vi "Example_Simple Acquire.vi"() -> ()   [LabVIEW 2015, in "G 5.lvlib"]
uses:
  <instrlib>/G 5.lvlib
  <vilib>/Utility/file.llb/Write To Spreadsheet File (DBL).vi
panel:
  in  "Display Duration [sec]":dbl=10.0
  in  "Acquisition Rate [Hz]":i16(ring)=2000 items=["10"=10, "15"=15, "20"=20, "25"=25, "30"=30, "40"=40, "45"=45, "50"=50, "60"=60, "75"=75, "80"=80, "90"=90, "100"=100, "120"=120, "125"=125, "150"=150, "180"=180, "200"=200, "225"=225, "240"=240, "250"=250, "300"=300, "360"=360, "400"=400, "450"=450, "500"=500, "600"=600, "800"=800, "900"=900, "1000"=1000, "1200"=1200, "1500"=1500, "1800"=1800, "2000"=2000]
  in  "Save Data":bool
  in  "Start Acquisition":bool
  in  "stop":bool
  in  "ZERO":bool
  in  "Gen 5":i32=1 min=1 step=1
  in  "CAPTURE":bool
  out "STATUS":bool=TRUE
  in  "Channel":i32=3
  in  "Value":dbl=5.0
  in  "Time [sec]":dbl=0.5 step=0.1 format="%.2g"
  out "Output Graph 2":waveform(dbl)[](graph)
  in  "Gen 5 Displayed 2":i64=2
  out "Output Graph 1":waveform(dbl)[](graph)
  in  "Gen 5 Displayed 1":i64=1
  # "TRIGGER CONTROL"
  # "ACQUISITION SETUP"
  # "ACQUISITION CONTROL"
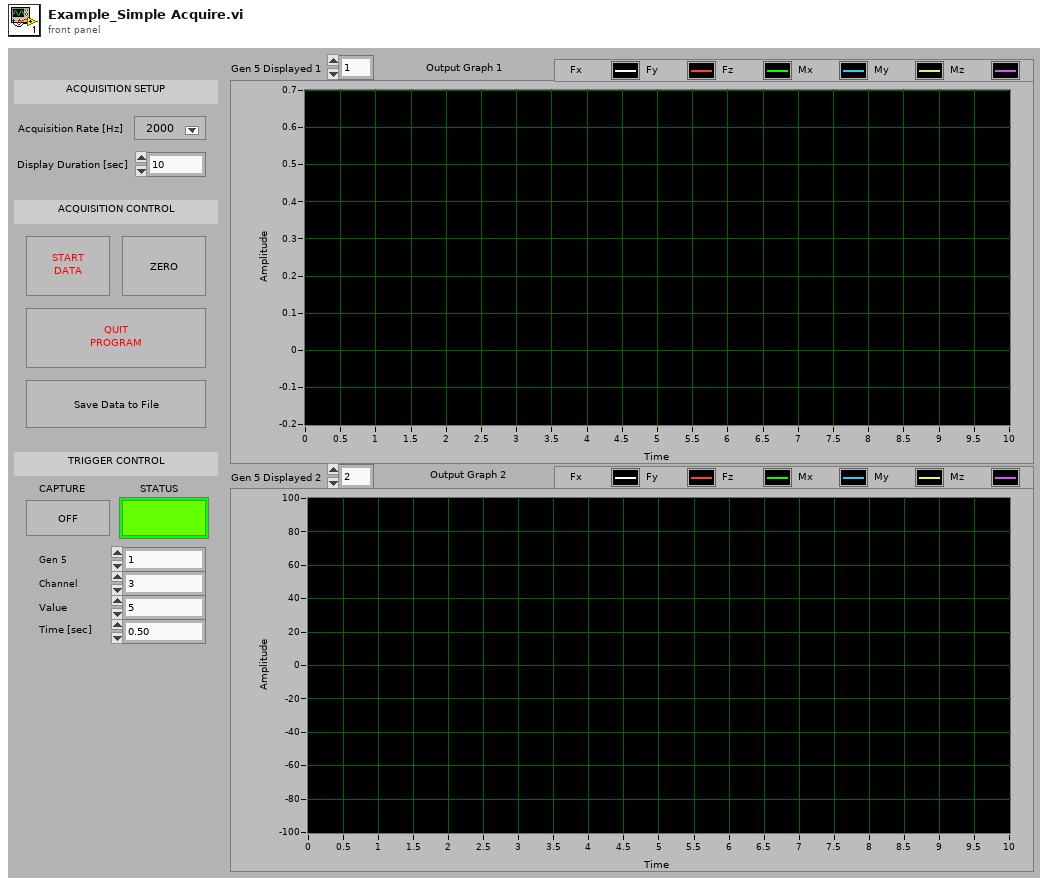
[diagram p1: front panel]
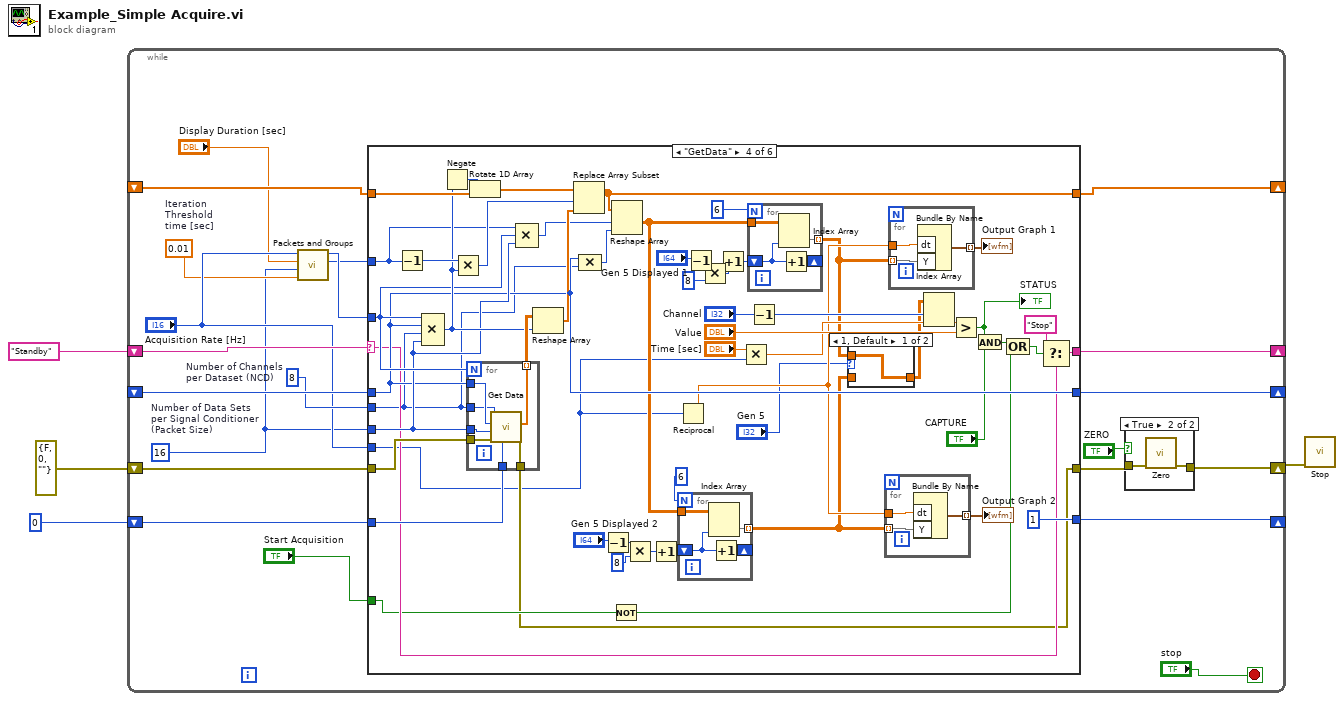
[diagram p0: block diagram]
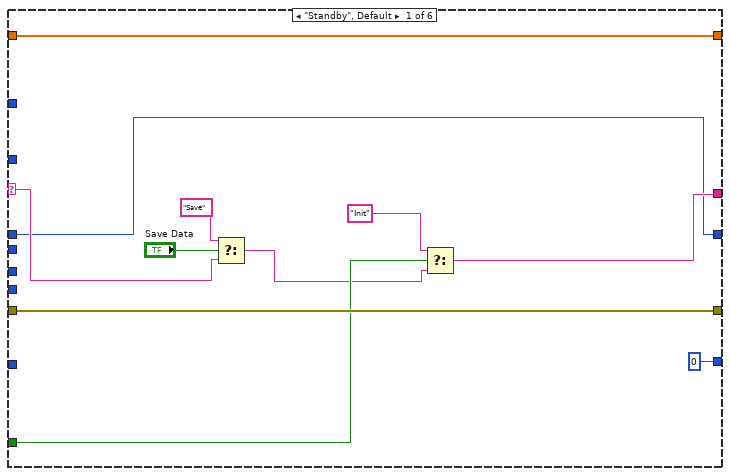
[diagram p3: hidden frame]
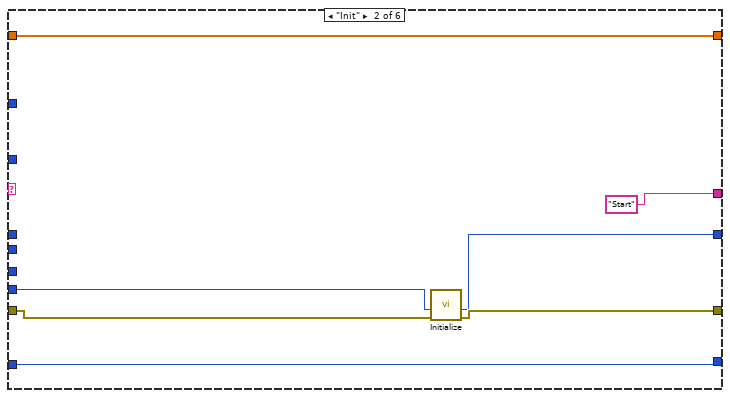
[diagram p4: hidden frame]
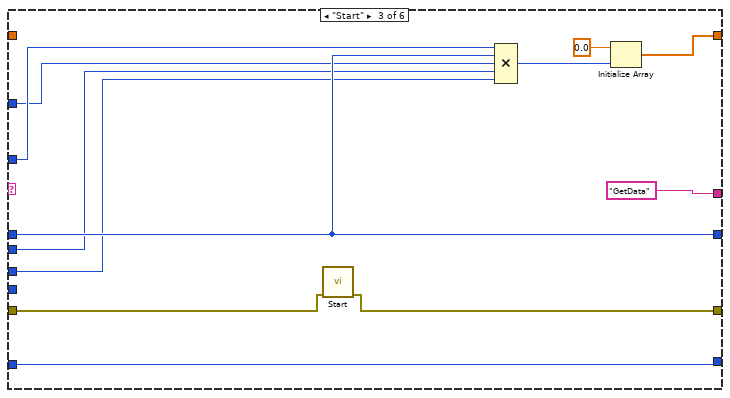
[diagram p5: hidden frame]
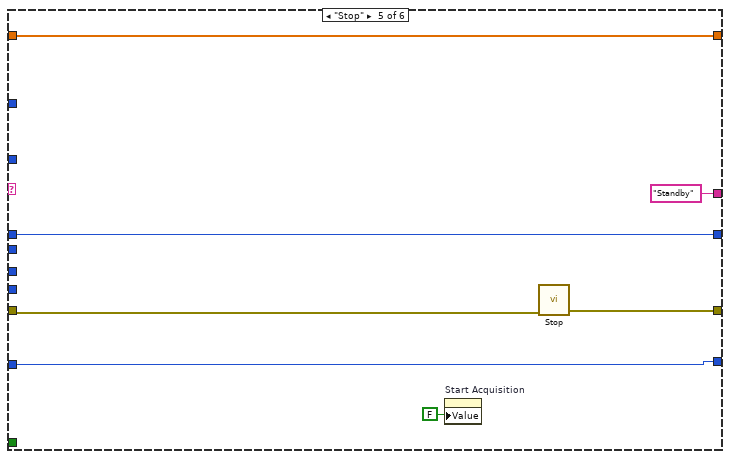
[diagram p7: hidden frame]
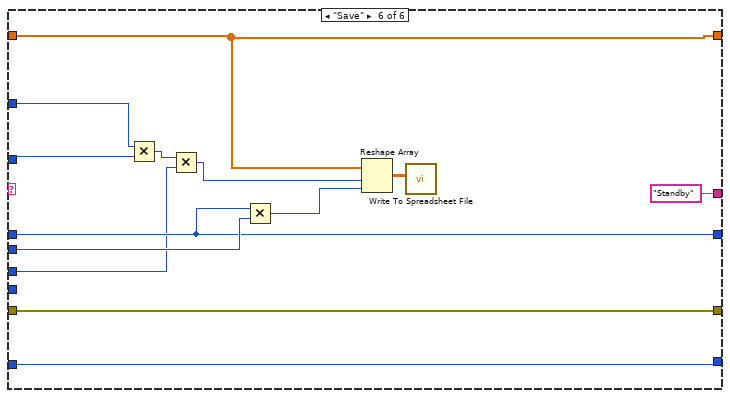
[diagram p8: hidden frame]
diagram:
  n1 = while {
    shift-right: [w20] -> _
    shift-left: "Standby" -> [w25]
    shift-right: [w23] -> w1
    shift-left: errorcluster {"status"=FALSE, "code"=0, "source"=""} ("error out") -> [w22]
    shift-right: [w19] -> _
    shift-left: _ -> [w18]
    shift-right: [w16] -> _
    shift-left: 0 -> [w17]
    shift-right: [w13] -> _
    shift-left: _ -> [w14]
    stop <- "stop" stop-if-true
    w9 = 0.01  # Iteration  Threshold  time [sec]
    w15 = 8  # Number of Channels per Dataset (NCD)
    w6 = 16  # Number of Data Sets  per Signal Conditioner (Packet Size)
    n2 = call <instrlib>:"Packets and Groups.vi"("Iteration Treshold Time [sec]"=w9, "Packet Size"=w6, "Duration [sec]"="Display Duration [sec]", "Acquisition Rate"="Acquisition Rate [Hz]") -> ("GROUPS"=w7:i32, "PACKETS"=w8:i32)  [unwired: 4 in, 2 out]
    n3 = case shown="\"GetData\"" w25 {
      selector: w25 -> [w32 _ _ w83 _ _]
      tunnel: w22 -> [w39 w46 w57 w112 w143 w154]
      tunnel: [w39 w45 w58 w76 w144 w154] -> w21
      tunnel: [w38 "Start" "GetData" w82 "Standby" "Standby"] -> w20
      tunnel: "Acquisition Rate [Hz]" -> [_ w43 _ w64 _ _]
      tunnel: [w29 w42 w51 w91 w141 w150] -> w19
      tunnel: w18 -> [w29 _ w51 w91 w141 w150]
      tunnel: w17 -> [_ w41 w47 w114 w140 w153]
      tunnel: [0 w41 w47 1 w140 w153] -> w16
      tunnel: w8 -> [_ _ w52 w99 _ w145]
      tunnel: w6 -> [_ _ w48 w98 _ w147]
      tunnel: w15 -> [_ _ w49 w79 _ w151]
      tunnel: w14 -> [w35 w40 _ w110 w139 w156]
      tunnel: w7 -> [_ _ w50 w100 _ w146]
      tunnel: [w35 w40 w54 w103 w139 w156] -> w13
      tunnel: "Start Acquisition" -> [w34 _ _ w80 _ _]
      frame "Standby", Default {
        n4 = Select(t="Save", s="Save Data", f=w32) -> (s? t:f=w31:string)
        n5 = Select(t="Init", s=w34, f=w31) -> (s? t:f=w38:string)
      }
      frame "Init" {
        n6 = call <instrlib>:"Initialize.vi"("error in (no error)"=w46, "Acquisition Rate"=w43) -> ("error out"=w45:errorcluster, "Device Count"=w42:i32)  [unwired: 8 in]
      }
      frame "Start" {
        n7 = call <instrlib>:"Start.vi"("error in (no error)"=w57) -> ("error out"=w58:errorcluster)  [unwired: 10 in]
        n8 = Compound Arithmetic op=MULTIPLY(w52, w51, w50, w49, w48) -> (w53:i32)
        n9 = Initialize Array(0.0 ("element"), w53) -> (w54:dbl[])
      }
      frame "GetData" {
        n10 = Decrement(x=w100) -> (x-1=w106:i32)
        n11 = Compound Arithmetic op=MULTIPLY(w99, w91, w79, w98) -> (w105:i32)
        n12 = Negate(x=w105) -> (-x=w109:i32)
        n13 = Multiply(x=w106, y=w105) -> (x*y=w104:i32)
        n14 = for {
          N: w99 -> [_]
          tunnel: w114 -> [w137]
          tunnel: [w133] -> w76
          tunnel: w91 -> [w134]
          tunnel: w112 -> [w136]
          tunnel: [w135] -> w111 mode=indexing
          tunnel: w98 -> [w132]
          tunnel: w79 -> [w131]
          n15 = call <instrlib>:"Get Data.vi"("Iteration"=w137, "error in"=w136, "N_DataSets\nper Gen5"=w132, "Device Count"=w134, "N_Channels\nper Dataset (NCD)"=w131) -> ("error out"=w133:errorcluster, "Data out"=w135:sgl[])  [unwired: 5 in]
        }
        n16 = Rotate 1D Array(1:w110, 2:w109) -> (0:w108:dbl[])
        n17 = Compound Arithmetic op=MULTIPLY(w100, w99, w98) -> (w102:i32)
        n18 = Reshape Array(w111, w105) -> (w107:sgl[])
        n19 = Replace Array Subset(array=w108, new element=w107, index=w104) -> (w103:dbl[])
        n20 = Compound Arithmetic op=MULTIPLY(w91, w79) -> (w101:i32)
        n21 = Decrement(x="Gen 5 Displayed 2") -> (x-1=w74:i64)
        n22 = Not(x=w80) -> (.not. x?=w67:bool)
        n23 = Reshape Array(w103, w102, w101) -> (w70:dbl[][])
        n24 = Multiply(x=w74, y=i64 8) -> (x*y=w73:i64)
        n25 = Increment(x=w73) -> (x+1=w72:i64)
        n26 = Reciprocal(x=w64) -> (1/x=w71:dbl)
        n27 = for {
          N: 6 -> [_]
          tunnel: w70 -> [w123]
          tunnel: [w122] -> w61 mode=indexing
          shift-right: [w121] -> _
          shift-left: w72 -> [w120]
          n28 = Index Array(array=w123, index (col)=w120) -> (element=w122:dbl[])  [unwired: 1 in]
          n29 = Increment(x=w120) -> (x+1=w121:i64)
        }
        n30 = Decrement(x="Gen 5 Displayed 1") -> (x-1=w95:i64)
        n31 = Multiply(x=w95, y=i64 8) -> (x*y=w93:i64)
        n32 = Increment(x=w93) -> (x+1=w69:i64)
        n33 = Multiply(x="Time [sec]", y=w64) -> (x*y=w78:dbl)
        n34 = for {
          N: 6 -> [_]
          tunnel: w70 -> [w130]
          tunnel: [w129] -> w60 mode=indexing
          shift-right: [w128] -> _
          shift-left: w69 -> [w127]
          n35 = Index Array(array=w130, index (col)=w127) -> (element=w129:dbl[])  [unwired: 1 in]
          n36 = Increment(x=w127) -> (x+1=w128:i64)
        }
        n37 = Decrement(x="Channel") -> (x-1=w87:i32)
        n38 = case shown="1, Default" "Gen 5" {
          tunnel: w61 -> [_ w116]
          tunnel: w60 -> [w115 _]
          tunnel: [w115 w116] -> w59
          frame 1, Default {
          }
          frame 2 {
          }
        }
        n39 = for {
          tunnel: [w119] -> w65 mode=indexing
          tunnel: w61 -> [w118] mode=indexing
          tunnel: w71 -> [w117]
          n40 = Bundle By Name("dt"=w117, "Y"=w118) -> (w119:waveform(dbl))  [unwired: 1 in]
        }
        "Output Graph 2" <- w65
        n41 = for {
          tunnel: [w126] -> w92 mode=indexing
          tunnel: w60 -> [w125] mode=indexing
          tunnel: w71 -> [w124]
          n42 = Bundle By Name("dt"=w124, "Y"=w125) -> (w126:waveform(dbl))  [unwired: 1 in]
        }
        "Output Graph 1" <- w92
        n43 = Index Array(array=w59, index (row)=w87, index (col)=w78) -> (element=w89:dbl)
        n44 = Greater?(x=w89, y="Value") -> (0:w84:bool)
        "STATUS" <- w84
        n45 = And(x=w84, y="CAPTURE") -> (x .and. y?=w68:bool)
        n46 = Compound Arithmetic op=OR(w68, w67) -> (w66:bool)
        n47 = Select(t="Stop", s=w66, f=w83) -> (s? t:f=w82:string)
      }
      frame "Stop" {
        n48 = property on="Start Acquisition" class="Bool (strict)"("Value"=FALSE ("Start Acquisition")) -> ()  [unwired: 2 in, 2 out]
        n49 = call <instrlib>:"Stop.vi"("error in (no error)"=w143) -> ("error out"=w144:errorcluster)  [unwired: 10 in]
      }
      frame "Save" {
        n50 = Multiply(x=w146, y=w145) -> (x*y=w148:i32)
        n51 = Multiply(x=w148, y=w147) -> (x*y=w149:i32)
        n52 = Multiply(x=w150, y=w151) -> (x*y=w152:i32)
        n53 = Reshape Array(w156, w149, w152) -> (w157:dbl[][])
        n54 = call-poly <vilib>:"Write To Spreadsheet File.vi"("2D data"=w157) -> ()  [unwired: 7 in, 1 out]
      }
    }
    n55 = case shown="True" "ZERO" {
      tunnel: w21 -> [w26 w28]
      tunnel: [w26 w27] -> w23
      frame False {
      }
      frame True {
        n56 = call <instrlib>:"Zero.vi"("error in (no error)"=w28) -> ("error out"=w27:errorcluster)  [unwired: 10 in]
      }
    }
  }
  n57 = call <instrlib>:"Stop.vi"("error in (no error)"=w1) -> ()  [unwired: 10 in, 1 out]
